vi "Test Confluence VIDoc.vi"() -> ()   [LabVIEW 2023]
uses:
  Source/Documentation Generation/Classes/Progress Bar UI/Progress Bar UI.lvclass
  C:/projects/DMC/GitHub/DMC CLI VIDoc/Source/Documentation Generation/UI Interaction/UI Interaction.lvclass
  Source/Documentation Generation/Printers/Confluence Printer/VIDoc Printer - Confluence.lvclass
  C:/projects/DMC/GitHub/DMC CLI VIDoc/Source/Documentation Generation/Classes/Progress Bar UI/Progress Bar UI.lvclass
  Source/Documentation Generation/Parsing/Documentation Parser/VIDoc Parser.lvclass
panel:
  in  "Top Page ID":string
  in  "Git History?":bool
  in  "Source Root":path
  in  "VIDoc json Settings Path":path
  out "Group":string
  out "Section":string
  out "error out":errorcluster {"code" format="Error %.0f"}
  out "Message":string
  out "Progress Bar":i32(slide) max=28 scale=0.0..18.0
  in  "Abort":bool
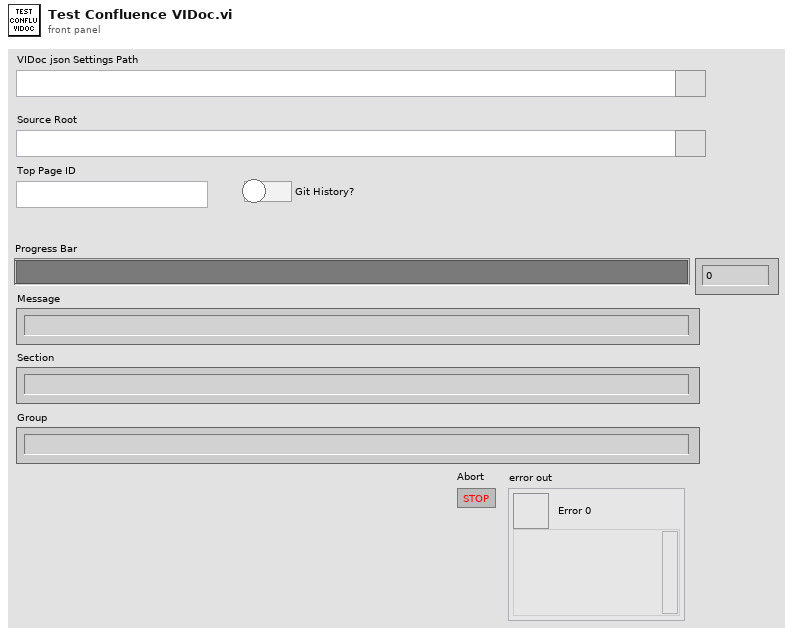
[diagram p1: front panel]
types:
  T1 = cluster{"Progress Max":refnum<user-event>, "Progress Value":refnum<user-event>, "Message":refnum<user-event>, "Stopped":refnum<user-event>, "Section":refnum<user-event>, "Group":refnum<user-event>}
  T2 = typedef "File Change Map.ctl" = map{string, cluster{"Timestamp":timestamp, "Commit Hash":string, "Author Name":string, "Branch":string, "Commit Hash URL":string}}
  T3 = typedef "VIDoc Parsing.lvlib/Full Documentation Info.ctl" = cluster{"Projects":refnum<class "Project Documentation.lvclass">[], "Interfaces":refnum<class "Interface Documenation.lvclass">[], "Classes":refnum<class "Class Documentation.lvclass">[], "Libraries":refnum<class "Library Documentation.lvclass">[], "GUIs":refnum<class "GUI Documentation.lvclass">[], "SubPanels":refnum<class "GUI Documentation.lvclass">[], "Dialogs":refnum<class "GUI Documentation.lvclass">[], "VI Members":refnum<class "GUI Documentation.lvclass">[], "Controls":refnum<class "GUI Documentation.lvclass">[], "LLBs":refnum<class "LLB Documentation.lvclass">[]}
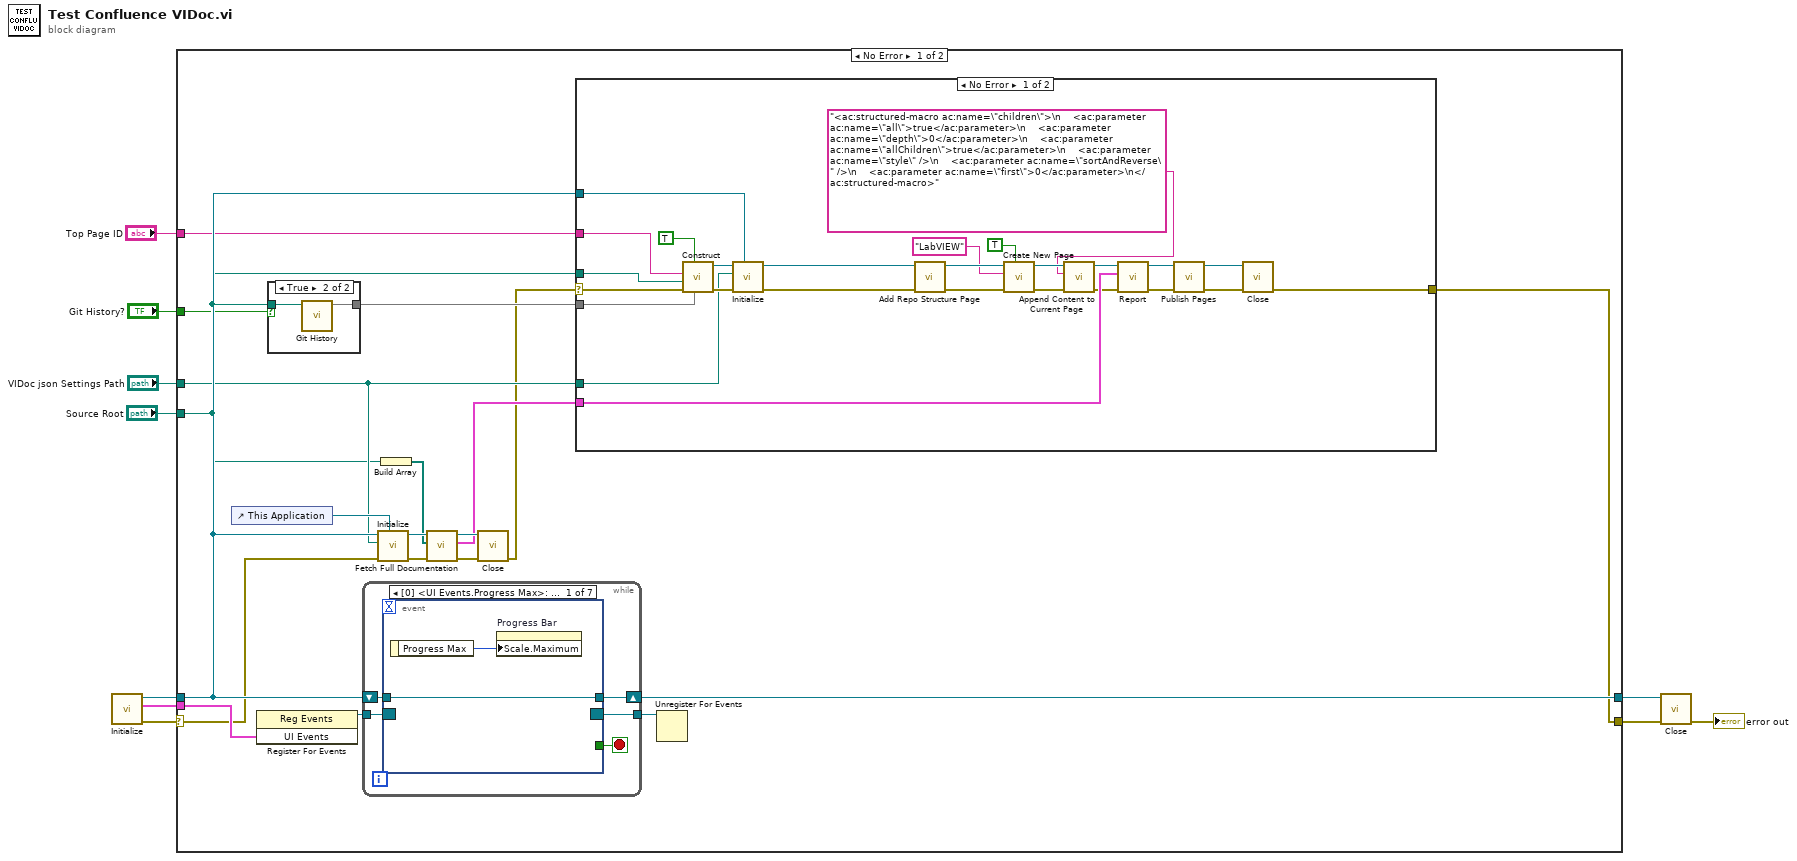
[diagram p0: block diagram]
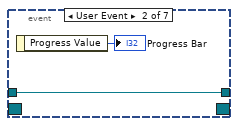
[diagram p3: hidden frame]
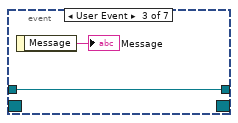
[diagram p4: hidden frame]
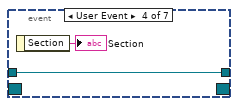
[diagram p5: hidden frame]
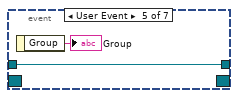
[diagram p6: hidden frame]
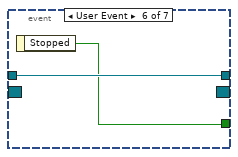
[diagram p7: hidden frame]
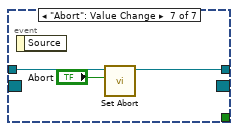
[diagram p8: hidden frame]
diagram:
  n1 = call "Initialize.vi"() -> ("error out"=w7:errorcluster, "UI Events"=w10:T1, "Progress Bar UI Out"=w8:refnum<class "Progress Bar UI.lvclass">)  [unwired: 9 in]
  n2 = case shown="No Error" w7 {
    selector: w7 -> [w17 w81]
    tunnel: w10 -> [w30 _]
    tunnel: [w28 w80] -> w9
    tunnel: w8 -> [w27 w80]
    tunnel: [w22 w81] -> w6
    tunnel: "VIDoc json Settings Path" -> [w16 _]
    tunnel: "Source Root" -> [w15 _]
    tunnel: "Git History?" -> [w14 _]
    tunnel: "Top Page ID" -> [w13 _]
    frame No Error {
      n3 = control-ref of="This Application"() -> (w19:refnum<vi>)
      n4 = register-events(w30) -> (reference out=w29:refnum<event-registration>)  [unwired: 2 in, 1 out]
      n5 = case shown="True" w14 {
        tunnel: [_ w79] -> w18
        tunnel: w15 -> [_ w78]
        frame False {
        }
        frame True {
          n6 = call "Git History.vi"("Working Directory"=w78) -> ("File Change Map"=w79:T2)  [unwired: 9 in, 1 out]
        }
      }
      n7 = while {
        tunnel: w29 -> [w62]
        shift-right: [w60] -> w28
        shift-left: w27 -> [w61]
        tunnel: [w58] -> w12
        stop <- w59 stop-if-true
        n8 = event shown="[0] <UI Events.Progress Max>: User Event" {
          selector: w62 -> [_ _ _ _ _ _ _]
          dyn-events: [_ _ _ _ _ _ _] -> w58
          timeout: _ -> [_ _ _ _ _ _ _]
          tunnel: w61 -> [w64 w66 w68 w70 w72 w74 w76]
          tunnel: [w64 w66 w68 w70 w72 w74 w77] -> w60
          tunnel: [_ _ _ _ _ w73 _] -> w59
          event User Event {
            n9 = event-data() -> ("Progress Max"=w63:i32)  [unwired: 1 in]
            n10 = property on="Progress Bar" class="Slide (strict)"("Scale.Maximum"=w63) -> ()  [unwired: 2 in, 2 out]
          }
          event User Event {
            n11 = event-data() -> ("Progress Value"=→"Progress Bar":i32)  [unwired: 1 in]
          }
          event User Event {
            n12 = event-data() -> ("Message"=→"Message":string)  [unwired: 1 in]
          }
          event User Event {
            n13 = event-data() -> ("Section"=→"Section":string)  [unwired: 1 in]
          }
          event User Event {
            n14 = event-data() -> ("Group"=→"Group":string)  [unwired: 1 in]
          }
          event User Event {
            n15 = event-data() -> ("Stopped"=w73:bool)  [unwired: 1 in]
          }
          event "Abort": Value Change {
            n16 = event-data() -> ()  [unwired: 1 in, 1 out]
            n17 = call "Set Abort.vi"("Abort?"="Abort", "Progress Bar UI In"=w76) -> ("Progress Bar UI Out"=w77:refnum<class "Progress Bar UI.lvclass">)  [unwired: 8 in, 1 out]
          }
        }
      }
      n18 = call "Initialize.vi"("App Reference (This Application)"=w19, "error in (no error)"=w17, "Settings Path"=w16, "UI Interaction"=w27) -> ("error out"=w26:errorcluster, "VIDoc Parser Out"=w25:refnum<class "VIDoc Parser.lvclass">)  [unwired: 6 in]
      n19 = Build Array(w15) -> (w20:path[])
      n20 = call "Fetch Full Documentation.vi"("error in (no error)"=w26, "File Paths"=w20, "VIDoc Parser In"=w25) -> ("error out"=w23:errorcluster, "Full Documentation"=w21:T3, "VIDoc Parser Out"=w24:refnum<class "VIDoc Parser.lvclass">)  [unwired: 6 in]
      n21 = call "Close.vi"("error in (no error)"=w23, "VIDoc Parser In"=w24) -> ("error out"=w11:errorcluster)  [unwired: 9 in]
      n22 = case shown="No Error" w11 {
        selector: w11 -> [w31 w57]
        tunnel: w27 -> [w56 _]
        tunnel: [w55 w57] -> w22
        tunnel: w21 -> [w54 _]
        tunnel: w18 -> [w46 _]
        tunnel: w16 -> [w45 _]
        tunnel: w15 -> [w44 _]
        tunnel: w13 -> [w43 _]
        frame No Error {
          n23 = call "Construct.vi"("File Change Map"=w46, "Bulk Attachments? (T)"=TRUE, "error in (no error)"=w31, "Working Directory"=w44, "Top Page ID"=w43) -> ("error out"=w53:errorcluster, "VIDoc Printer - Confluence Out"=w52:refnum<class "VIDoc Printer - Confluence.lvclass">)  [unwired: 5 in]
          n24 = call-dynamic "Initialize.vi"("UI Interaction"=w56, "error in (no error)"=w53, "Settings Path"=w45, "VIDoc Printer - Confluence In"=w52) -> ("error out"=w51:errorcluster, "VIDoc Printer - Confluence Out"=w50:refnum<class "VIDoc Printer - Confluence.lvclass">)  [unwired: 6 in]
          n25 = call "Add Repo Structure Page.vi"("error in (no error)"=w51, "VIDoc Printer - Confluence In"=w50) -> ("error out"=w40:errorcluster, "VIDoc Printer - Confluence Out"=w39:refnum<class "VIDoc Printer - Confluence.lvclass">)  [unwired: 8 in]
          n26 = call "Create New Page.vi"("Update Current Page (F)"=TRUE, "error in (no error)"=w40, "Name"="LabVIEW", "VIDoc Printer - Confluence In"=w39) -> ("error out"=w34:errorcluster, "VIDoc Printer - Confluence Out"=w36:refnum<class "VIDoc Printer - Confluence.lvclass">)  [unwired: 4 in, 2 out]
          n27 = call "Append Content to Current Page.vi"("error in (no error)"=w34, "Content"="<ac:structured-macro ac:name=\"children\">\n    <ac:parameter ac:name=\"all\">true</ac:parameter>\n    <ac:parameter ac:name=\"depth\">0</ac:parameter>\n    <ac:parameter ac:name=\"allChildren\">true</ac:parameter>\n    <ac:parameter ac:name=\"style\" />\n    <ac:parameter ac:name=\"sortAndReverse\" />\n    <ac:parameter ac:name=\"first\">0</ac:parameter>\n</ac:structured-macro>", "VIDoc Printer - Confluence In"=w36) -> ("error out"=w33:errorcluster, "VIDoc Printer - Confluence Out"=w35:refnum<class "VIDoc Printer - Confluence.lvclass">)  [unwired: 7 in]
          n28 = call-dynamic "Report.vi"("error in (no error)"=w33, "Full Documentation"=w54, "VIDoc Printer In"=w35) -> ("error out"=w42:errorcluster, "VIDoc Printer Out"=w41:refnum<class "VIDoc Printer - Confluence.lvclass">)  [unwired: 7 in]
          n29 = call "Publish Pages.vi"("error in (no error)"=w42, "VIDoc Printer - Confluence In"=w41) -> ("error out"=w48:errorcluster, "VIDoc Printer - Confluence Out"=w47:refnum<class "VIDoc Printer - Confluence.lvclass">)  [unwired: 8 in]
          n30 = call-dynamic "Close.vi"("error in (no error)"=w48, "VIDoc Printer - Confluence In"=w47) -> ("error out"=w55:errorcluster)  [unwired: 9 in]
        }
        frame Error {
        }
      }
      n31 = Unregister For Events(event registration refnum=w12) -> ()  [unwired: 1 in, 1 out]
    }
    frame Error {
    }
  }
  n32 = call "Close.vi"("error in (no error)"=w6, "Progress Bar UI In"=w9) -> ("error out"=→"error out":errorcluster)  [unwired: 9 in]
